vi "E3631A Configuration Output.vi"(5 "Enable Output (T: Enable)":bool=TRUE, 7 "Channel (1: Channel 1)":i32(ring)=1 items=["Channel 1"=1, "Channel 2"=2, "Channel 3"=3], 8 "error in (no error)":errorcluster, 10 "Voltage Level (0.0 V)":dbl format="%.3g", 11 "VISA resource name":refnum<visa-resource-name>) -> (0 "error out":errorcluster, 3 "VISA resource name out":refnum<visa-resource-name>)   [LabVIEW 2017]
panel:
  out "resulting string":string
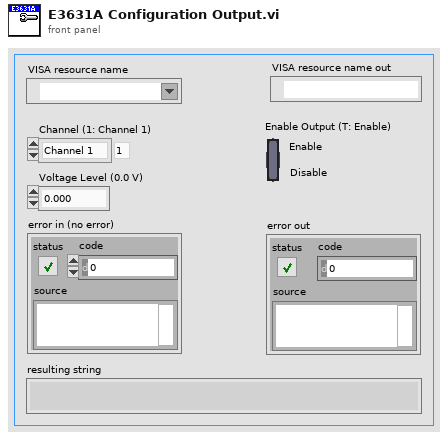
[diagram p1: front panel]
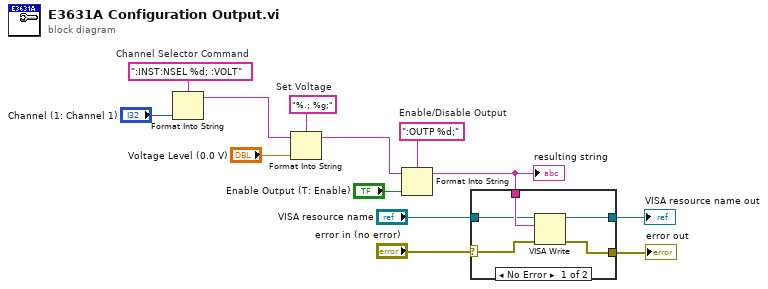
[diagram p0: block diagram]
diagram:
  w9 = ":OUTP %d;"  # Enable/Disable Output
  w11 = "%.; %g;"  # Set Voltage
  w13 = ":INST:NSEL %d; :VOLT"  # Channel Selector Command
  n1 = Format Into String(format string=w13, "Channel (1: Channel 1)") -> (resulting string=w7:string)  [unwired: 2 in, 1 out]
  n2 = Format Into String(format string=w11, initial string=w7, "Voltage Level (0.0 V)") -> (resulting string=w6:string)  [unwired: 1 in, 1 out]
  n3 = Format Into String(format string=w9, initial string=w6, "Enable Output (T: Enable)") -> (resulting string=w5:string)  [unwired: 1 in, 1 out]
  "resulting string" <- w5
  n4 = case shown="No Error" "error in (no error)" {
    selector: "error in (no error)" -> [w14 w20]
    tunnel: w5 -> [w18 _]
    tunnel: "VISA resource name" -> [w17 w19]
    tunnel: [w16 w19] -> w3
    tunnel: [w15 w20] -> w2
    frame No Error {
      n5 = VISA Write(VISA resource name=w17, write buffer=w18, error in (no error)=w14) -> (VISA resource name out=w16:refnum<visa-resource-name>, error out=w15:errorcluster)  [unwired: 1 out]
    }
    frame Error {
    }
  }
  "VISA resource name out" <- w3
  "error out" <- w2
